vi "TempLog.vi"() -> ()   [LabVIEW 2010]
uses:
  <instrlib>/Agilent 34401/Public/Data/Read (Single Point).vi
  <instrlib>/Agilent 34401/Agilent 34401.lvlib
panel:
  out "Last value time":string
  out "Waveform Chart":dbl(graph)
  out "error out":errorcluster
  in  "stop":bool
  out "Last value":dbl format="%#_10p"
  in  "VISA resource name":refnum<visa-resource-name>
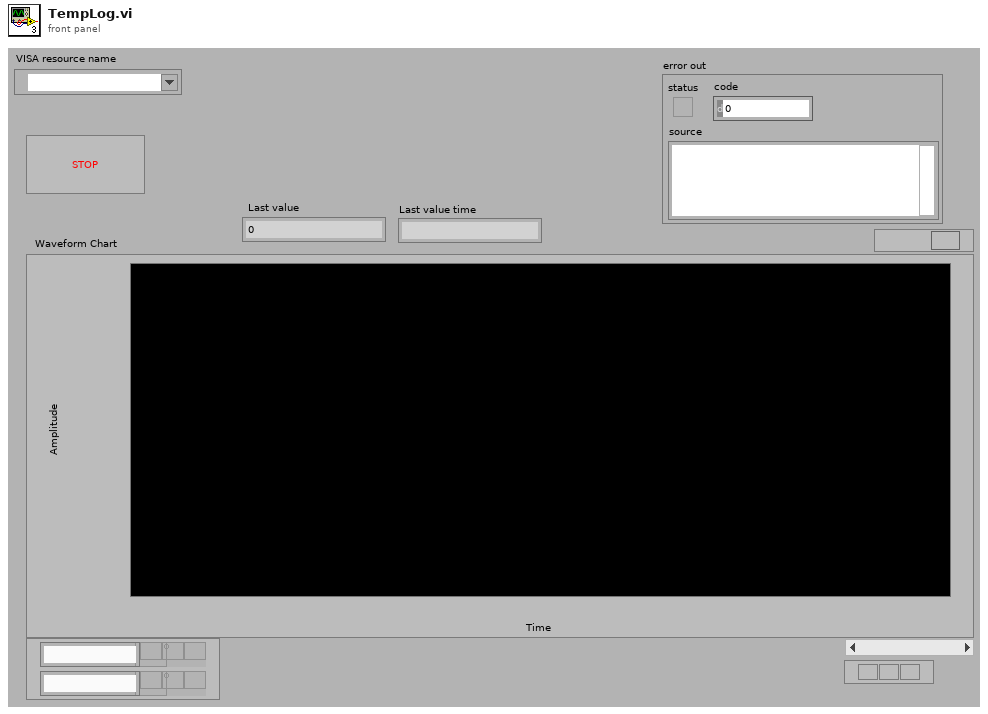
[diagram p1: front panel]
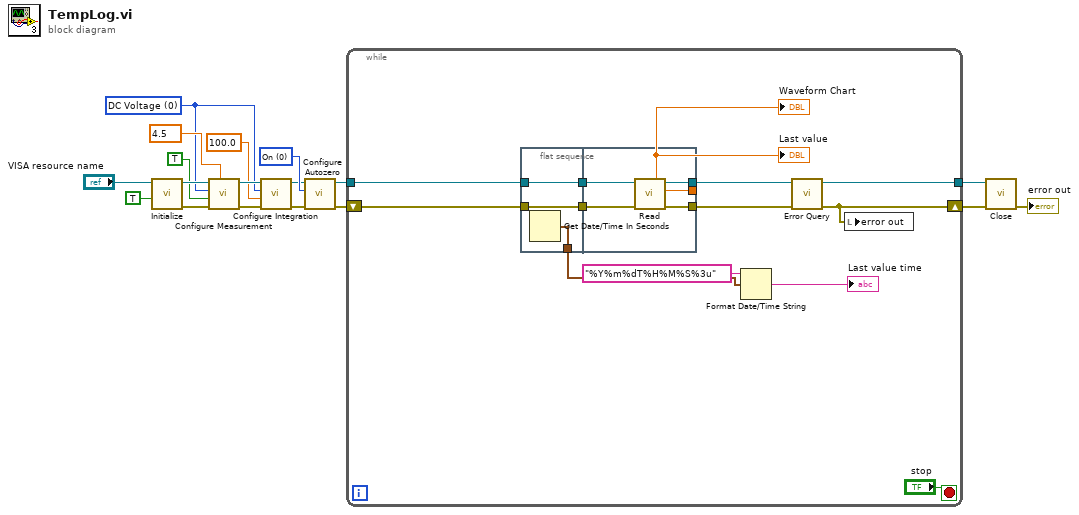
[diagram p0: block diagram]
diagram:
  w2 = u16 0 items=["On", "Off", "Once"] ("Autozero  (0: On)")
  w4 = 100.0 items=["0.001"=0.001, "0.002"=0.002, "0.006"=0.006, "0.02"=0.02, "0.06"=0.06, "0.2"=0.2, "1"=1.0, "10"=10.0, "100"=100.0] ("Integration Time (1 PLCs)")
  w8 = 4.5 items=["4.5"=4.5, "5.5"=5.5, "6.5"=6.5] ("Manual Resolution (5.5 Digits)")
  w7 = u16 0 items=["DC Voltage", "AC Voltage", "2 - Wire Resistance", "4 - Wire Resistance", "DC Current", "AC Current", "Frequency", "Period", "Continuity", "Diode Checking", "VDC:VDC Ratio", "Temperature", "Capacitance"] ("Function (0: DC Voltage)")
  n1 = call <instrlib>:"Initialize.vi"("Reset (True)"=TRUE, "VISA resource name"="VISA resource name") -> ("error out"=w11:errorcluster, "VISA resource name out"=w12:refnum<visa-resource-name>)  [unwired: 8 in]
  n2 = call <instrlib>:"Configure Measurement.vi"("Manual Resolution (5.5 Digits)"=w8, "error in (no error)"=w11, "Enable Auto Range (T: Enable)"=TRUE, "Function (0: DC Voltage)"=w7, "VISA resource name"=w12) -> ("error out"=w10:errorcluster, "VISA resource name out"=w9:refnum<visa-resource-name>)  [unwired: 5 in]
  n3 = call <instrlib>:"Configure Integration.vi"("error in (no error)"=w10, "Integration Time (1 PLCs)"=w4, "Function (0: DC Voltage)"=w7, "VISA resource name"=w9) -> ("error out"=w3:errorcluster, "VISA resource name out"=w1:refnum<visa-resource-name>)  [unwired: 6 in]
  n4 = call <instrlib>:"Configure Autozero.vi"("error in (no error)"=w3, "Autozero  (0: On)"=w2, "VISA resource name"=w1) -> ("error out"=w16:errorcluster, "VISA resource name out"=w17:refnum<visa-resource-name>)  [unwired: 7 in]
  n5 = while {
    tunnel: w17 -> [w27]
    shift-right: [w30] -> w14
    shift-left: w16 -> [w28]
    tunnel: [w29] -> w15
    stop <- "stop" stop-if-true
    n6 = flat-sequence {
      tunnel: w27 -> [w33]
      tunnel: w28 -> [w34]
      tunnel: [w34] -> w23
      tunnel: [w33] -> w22
      tunnel: [w32] -> w21
      tunnel: [w37] -> w26
      tunnel: [w36] -> w25
      tunnel: [w35] -> w24
      tunnel: w23 -> [w39]
      tunnel: w22 -> [w38]
      frame #0 {
        n7 = Get Date/Time In Seconds() -> (seconds since 1Jan1904=w32:timestamp)
      }
      frame #1 {
        n8 = call-poly <instrlib>:"Read.vi"("error in (no error)"=w39, "VISA resource name"=w38) -> ("error out"=w35:errorcluster, "Measurement"=w36:dbl, "VISA resource name out"=w37:refnum<visa-resource-name>)  [unwired: 7 in]
      }
    }
    n9 = Format Date/Time String(time format string (%c)="%Y%m%dT%H%M%S%3u", seconds (now)=w21) -> (date/time string=→"Last value time":string)  [unwired: 1 in]
    n10 = call <instrlib>:"Error Query.vi"("error in (no error)"=w24, "VISA resource name"=w26) -> ("error out"=w30:errorcluster, "VISA resource name out"=w29:refnum<visa-resource-name>)  [unwired: 6 in, 2 out]
    n11 = local write "error out"(w30) -> ()
    "Last value" <- w25
    "Waveform Chart" <- w25
  }
  n12 = call <instrlib>:"Close.vi"("error in (no error)"=w14, "VISA resource name"=w15) -> ("error out"=→"error out":errorcluster)  [unwired: 9 in]
